vi "cal_sub_ring_const_pos.vi"(0 "BD Text":string, 5 "1st sub node x position":i32, 7 "Last Function Position":cluster{"Left":i32, "Top":i32}, 9 "Last Control Position":cluster{"Left":i32, "Top":i32}, 11 "error in":errorcluster) -> (6 "BD Node Position":cluster{"1st sub node x position":i32, i32}, 10 "BD Constant Position":cluster{i32, i32}, 15 "error out":errorcluster)   [LabVIEW 2018]
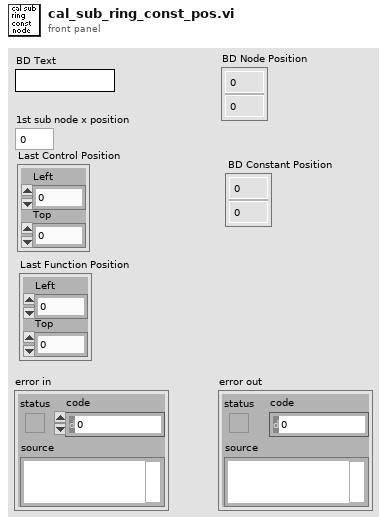
[diagram p1: front panel]
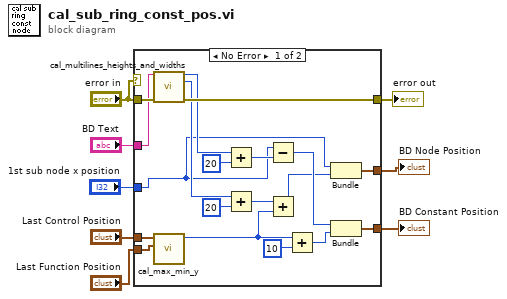
[diagram p0: block diagram]
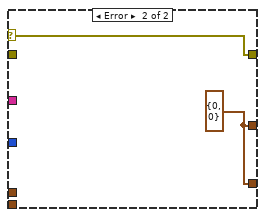
[diagram p2: hidden frame]
diagram:
  n1 = case shown="No Error" "error in" {
    selector: "error in" -> [_ w29]
    tunnel: [w27 w29] -> w8
    tunnel: "error in" -> [w26 _]
    tunnel: "BD Text" -> [w18 _]
    tunnel: [w17 w28] -> w6
    tunnel: "1st sub node x position" -> [w15 _]
    tunnel: [w12 w28] -> w4
    tunnel: "Last Control Position" -> [w11 _]
    tunnel: "Last Function Position" -> [w10 _]
    frame No Error {
      n2 = call "cal_multilines_heights_and_widths.vi"("Ring Command"=w18, "error in (no error)"=w26) -> ("BD Width"=w19:i32, "BD Height"=w16:i32, "error out"=w27:errorcluster)  [unwired: 4 in, 7 out]
      n3 = call "cal_max_min_y.vi"("Position 2"=w10, "Position 1"=w11) -> ("max y"=w9:i32)  [unwired: 9 out]
      n4 = Add(x=w19, y=20) -> (x+y=w21:i32)
      n5 = Add(x=w16, y=20) -> (x+y=w13:i32)
      n6 = Subtract(x=w15, y=w21) -> (x-y=w22:i32)
      n7 = Add(x=w13, y=w9) -> (x+y=w14:i32)
      n8 = Add(x=w9, y=10) -> (x+y=w23:i32)
      n9 = Bundle("1st sub node x position"=w15, w14) -> (w12:cluster{"1st sub node x position":i32, i32})  [unwired: 1 out]
      n10 = Bundle(w22, w23) -> (w17:cluster{i32, i32})  [unwired: 1 out]
    }
    frame Error {
      w28 = cluster{i32, i32} {0, 0}
    }
  }
  "error out" <- w8
  "BD Constant Position" <- w6
  "BD Node Position" <- w4
